vi "Revision Query.vi"(8 "error in (no error)":errorcluster, 11 "VISA resource name":refnum<visa-resource-name>) -> (0 "error out":errorcluster, 2 "Instrument Driver Revision":string, 3 "VISA resource name out":refnum<visa-resource-name>)   [LabVIEW 2015, in "SR400.lvlib"]
doc: "Queries the current instrument firmware revision and instrument driver revision.\n\nRefer to the Readme file for detailed driver information including modification history."
uses:
  SR400.lvlib
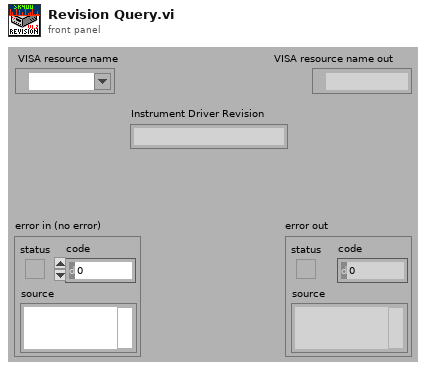
[diagram p1: front panel]
types:
  T1 = enum32{"invalid app kind", "Development System", "Run Time System", "Student Edition", "Embedded LabVIEW", "Evaluation", "Custom"}
  T2 = cluster{"Major":u16, "Minor":u16, "Fix":u16, "Build":u16}
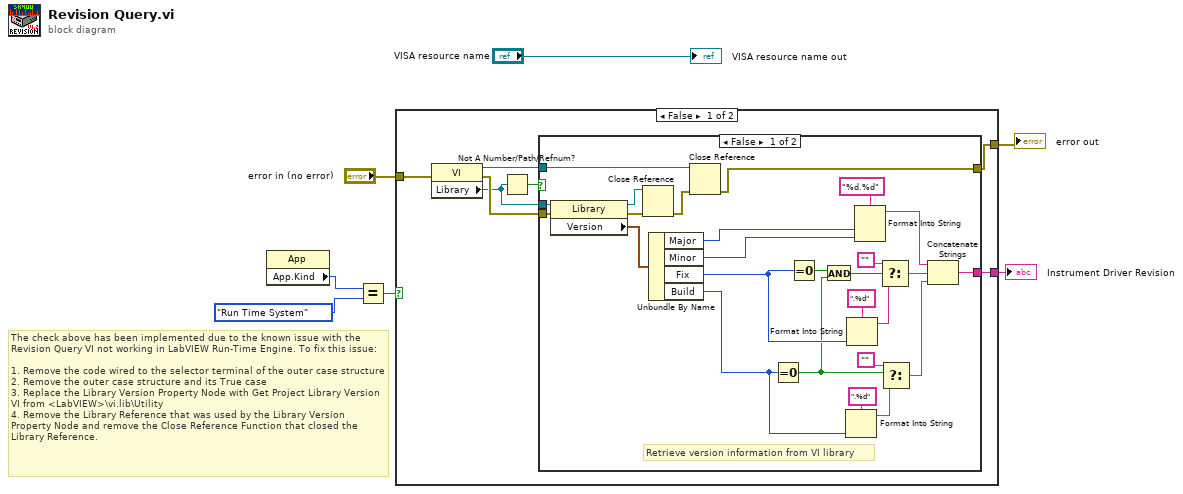
[diagram p0: block diagram]
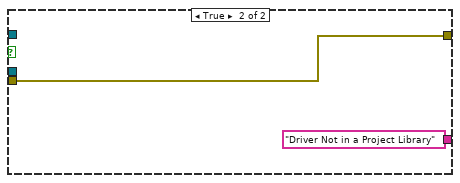
[diagram p2: hidden frame]
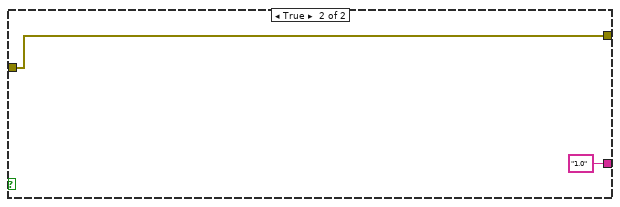
[diagram p3: hidden frame]
diagram:
  # "The check above has been implemented due to the known issue with the Revision Query VI not working in LabVIEW Run-Time Engine. To fix this issue:\n\n1. Remove the code wired to the selector terminal of the outer case structure\n2. Remove the outer case structure and its True case\n3. Replace the Library Version Property Node with Get Project Library Version VI from <LabVIEW>\\vi.lib\\Utility\n4. Remove the Library Reference that was used by the Library Version Property Node and remove the Close Reference Function that closed the Library Reference."
  n1 = property class="App"() -> ("App.Kind"=w4:T1)  [unwired: 2 in, 2 out]
  n2 = Equal?(x=w4, y=T1."Run Time System" ("Application:Kind")) -> (x = y?=w5:bool)
  n3 = case shown="False" w5 {
    tunnel: [w10 "1.0"] -> w7
    tunnel: "error in (no error)" -> [w9 w43]
    tunnel: [w8 w43] -> w1
    frame False {
      n4 = property class="VI"(error in=w9) -> (reference out=w14:refnum<vi>, error out=w13:errorcluster, "Library"=w12:refnum<vi>)  [unwired: 1 in]
      n5 = Not A Number/Path/Refnum?(number/path/refnum=w12) -> (NaN/Path/Refnum?=w11:bool)
      n6 = case shown="False" w11 {
        tunnel: w14 -> [w37 _]
        tunnel: w13 -> [w22 w42]
        tunnel: [w17 w42] -> w8
        tunnel: [w16 "Driver Not in a Project Library"] -> w10
        tunnel: w12 -> [w15 _]
        frame False {
          # "Retrieve version information from VI library"
          n7 = property class="Library"(reference=w15, error in=w22) -> (reference out=w39:refnum<vi>, error out=w40:errorcluster, "Version"=w36:T2)
          n8 = Close Reference(reference=w39, error in (no error)=w40) -> (error out=w38:errorcluster)
          n9 = Unbundle By Name(w36) -> ("Major"=w25:u16, "Minor"=w24:u16, "Fix"=w21:u16, "Build"=w23:u16)
          n10 = Close Reference(reference=w37, error in (no error)=w38) -> (error out=w17:errorcluster)
          n11 = Equal To 0?(x=w23) -> (x = 0?=w19:bool)
          n12 = Equal To 0?(x=w21) -> (x = 0?=w20:bool)
          n13 = And(x=w20, y=w19) -> (x .and. y?=w18:bool)
          n14 = Format Into String(format string=".%d", w23) -> (resulting string=w29:string)  [unwired: 2 in, 1 out]
          n15 = Format Into String(format string=".%d", w21) -> (resulting string=w33:string)  [unwired: 2 in, 1 out]
          n16 = Format Into String(format string="%d.%d", w25, w24) -> (resulting string=w31:string)  [unwired: 2 in, 1 out]
          n17 = Select(t="", s=w18, f=w33) -> (s? t:f=w30:string)
          n18 = Select(t="", s=w19, f=w29) -> (s? t:f=w26:string)
          n19 = Concatenate Strings(w31, w30, w26) -> (w16:string)
        }
        frame True {
        }
      }
    }
    frame True {
    }
  }
  "Instrument Driver Revision" <- w7
  "error out" <- w1
  "VISA resource name out" <- "VISA resource name"
